vi "PH-temp-raw.vi"(1 "array in":u32[](array[numeric]) format="%08x", 2 "command":string) -> (0 "array out":u32[](array[numeric]) format="%08x")   [LabVIEW 2015]
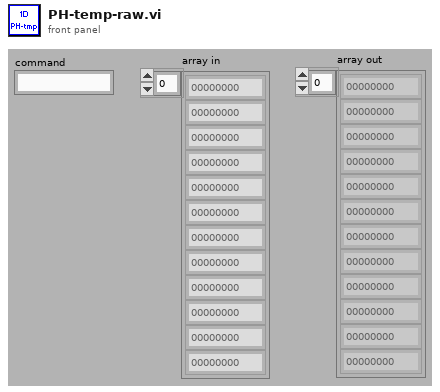
[diagram p1: front panel]
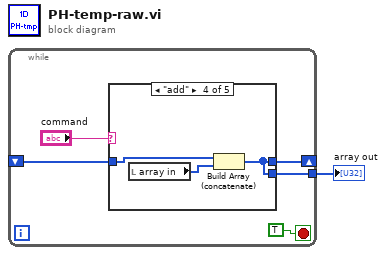
[diagram p0: block diagram]
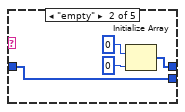
[diagram p3: hidden frame]
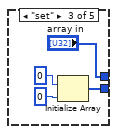
[diagram p4: hidden frame]
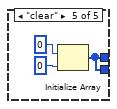
[diagram p5: hidden frame]
diagram:
  n1 = while {
    shift-right: [w2] -> _
    shift-left: _ -> [w5]
    tunnel: [w4] -> w1
    stop <- TRUE stop-if-true
    n2 = case shown="\"add\"" "command" {
      tunnel: [w7 w8 "array in" w16 w20] -> w2
      tunnel: w5 -> [w7 w11 _ w18 _]
      tunnel: [w7 w11 w14 w16 w20] -> w4
      frame "get", Default {
      }
      frame "empty" {
        n3 = Initialize Array(u32 0 ("element"), 0 ("dimension size")) -> (w8:u32[])
      }
      frame "set" {
        n4 = Initialize Array(u32 0 ("element"), 0 ("dimension size")) -> (w14:u32[])
      }
      frame "add" {
        n5 = local read "array in"() -> (w17:u32[])
        n6 = Build Array (concatenate)(w18, w17) -> (w16:u32[])
      }
      frame "clear" {
        n7 = Initialize Array(u32 0 ("element"), 0 ("dimension size")) -> (w20:u32[])
      }
    }
  }
  "array out" <- w1
